vi "Solve1.vi"(8 "Error In":errorcluster, 11 "object in":refnum<class "2025_1.lvclass">) -> (0 "Error Out":errorcluster, 2 "Result":u64, 3 "object out":refnum<class "2025_1.lvclass">)   [LabVIEW 2023, in "2025_1.lvclass"]
uses:
  2025_1.lvclass
  2025_1.lvclass/2025_1.ctl
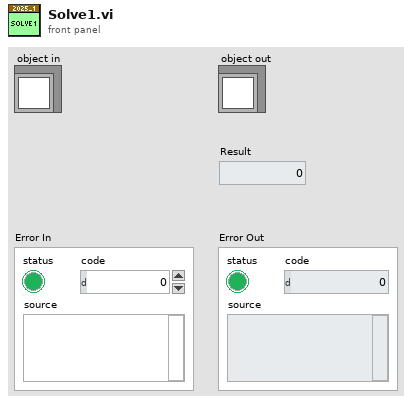
[diagram p1: front panel]
types:
  T1 = typedef "2025_1.lvclass/Turns.ctl" = cluster{"Direction":T2, "Steps":i64}
  T2 = typedef "2025_1.lvclass/Direction.ctl" = enum16{"Left", "Right"}
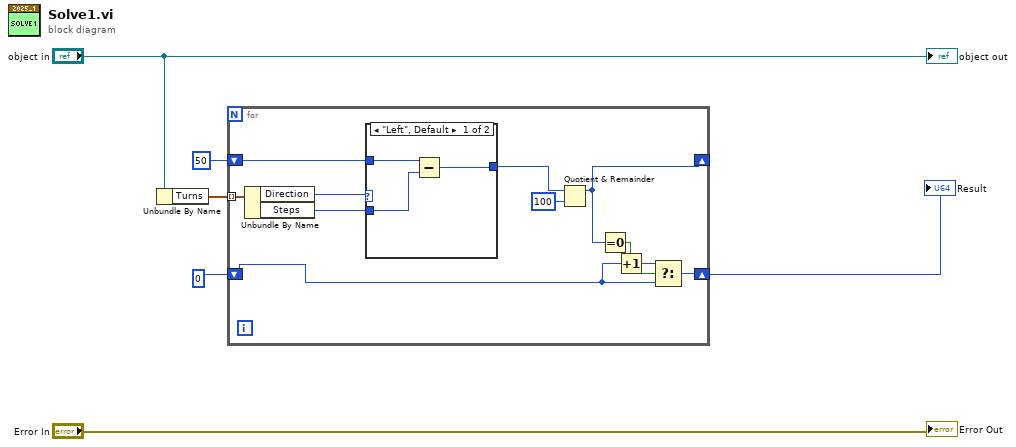
[diagram p0: block diagram]
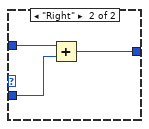
[diagram p2: hidden frame]
diagram:
  n1 = Unbundle By Name("object in") -> ("Turns"=w4:T1[])
  n2 = for {
    tunnel: w4 -> [w17] mode=indexing
    shift-right: [w7] -> _
    shift-left: i64 50 -> [w15]
    shift-right: [w11] -> w1
    shift-left: i64 0 -> [w10]
    n3 = Unbundle By Name(w17) -> ("Direction"=w16:T2, "Steps"=w14:i64)
    n4 = case shown="\"Left\", Default" w16 {
      tunnel: w15 -> [w20 w23]
      tunnel: [w18 w22] -> w8
      tunnel: w14 -> [w19 w21]
      frame "Left", Default {
        n5 = Subtract(x=w20, y=w19) -> (x-y=w18:i64)
      }
      frame "Right" {
        n6 = Add(x=w23, y=w21) -> (x+y=w22:i64)
      }
    }
    n7 = Quotient & Remainder(x=w8, y=i64 100) -> (x-y*floor(x/y)=w7:i64)  [unwired: 1 out]
    n8 = Equal To 0?(x=w7) -> (x = 0?=w12:bool)
    n9 = Increment(x=w10) -> (x+1=w9:i64)
    n10 = Select(t=w9, s=w12, f=w10) -> (s? t:f=w11:i64)
  }
  "Result" <- w1
  "Error Out" <- "Error In"
  "object out" <- "object in"
